vi "Read Convex Hull.vi"(8 "error in (no error)":errorcluster, 11 "Video Cam Processor in":refnum<class "Video Cam Processor.lvclass">) -> (0 "error out":errorcluster, 2 "Convex Hull":T1[][](array[typedef]), 3 "Video Cam Processor out":refnum<class "Video Cam Processor.lvclass">)   [LabVIEW 2018, in "Video Cam Processor.lvclass"]
uses:
  Video Cam Processor.lvclass
  Private/Hull Point STYP.ctl
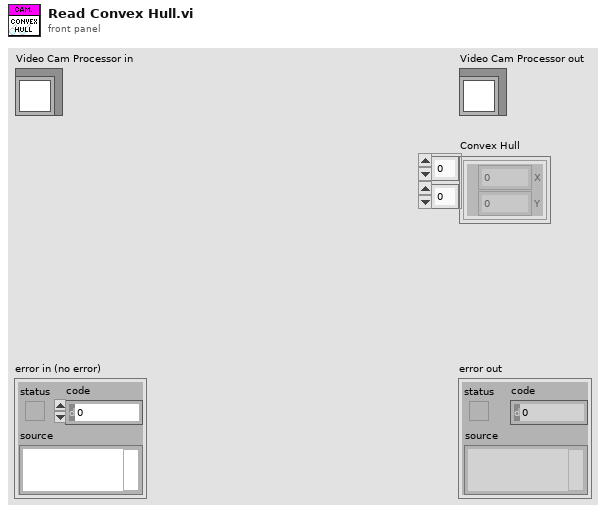
[diagram p1: front panel]
types:
  T1 = typedef "Video Cam Processor.lvclass/Hull Point STYP.ctl" = cluster{"X":i32, "Y":i32}
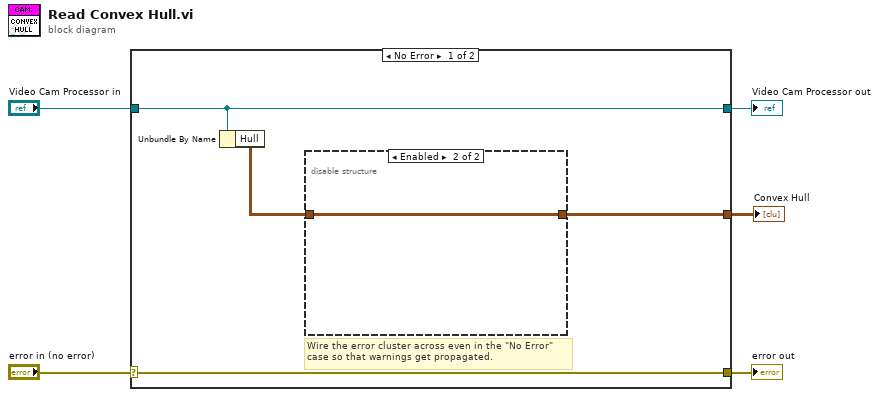
[diagram p0: block diagram]
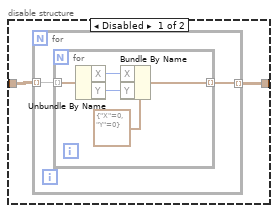
[diagram p2: hidden frame]
diagram:
  n1 = case shown="No Error" "error in (no error)" {
    selector: "error in (no error)" -> [w9 w21]
    tunnel: [w9 w21] -> w4
    tunnel: [w8 w20] -> w2
    tunnel: "Video Cam Processor in" -> [w8 w20]
    tunnel: [w6 _] -> w1
    frame No Error {
      # "Wire the error cluster across even in the \"No Error\"\ncase so that warnings get propagated."
      n2 = Unbundle By Name(w8) -> ("Hull"=w7:T1[][])
      n3 = disable-structure shown="Enabled" {
        disable-tunnel: w7 -> [w11 w19]
        disable-tunnel: [w10 w19] -> w6
        frame Disabled {
          n4 = for {
            tunnel: w11 -> [w13] mode=indexing
            tunnel: [w12] -> w10 mode=indexing
            n5 = for {
              tunnel: w13 -> [w18] mode=indexing
              tunnel: [w14] -> w12 mode=indexing
              n6 = Unbundle By Name(w18) -> ("X"=w16:i32, "Y"=w15:i32)
              n7 = Bundle By Name(cluster=T1 {"X"=0, "Y"=0} ("Cluster"), "X"=w16, "Y"=w15) -> (w14:T1)
            }
          }
        }
        frame Enabled {
        }
      }
    }
    frame Error {
    }
  }
  "error out" <- w4
  "Video Cam Processor out" <- w2
  "Convex Hull" <- w1
